vi "CalculateBPM.vi"(11 "Raw Beam Profile":dbl[][](array[numeric]) format="%0.2f") -> (3 "BPM":cluster{dbl[], "Beam Profile":dbl[]}[](array[cluster]))   [LabVIEW 2012]
uses:
  <vilib>/Analysis/_algsub.llb/Vector Norm Type.ctl
  <vilib>/Analysis/baseanly.llb/Normalize Vector.vi
  <vilib>/Analysis/baseanly.llb/Unit Vector (DBL).vi
  <vilib>/Analysis/NI_AALPro.lvlib
  <vilib>/Analysis/NI_AALBase.lvlib
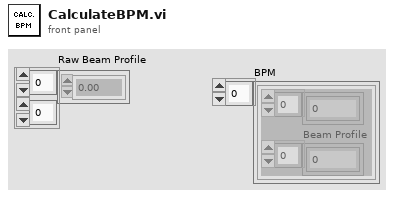
[diagram p1: front panel]
types:
  T1 = typedef "NI_AALPro.lvlib/Vector Norm Type.ctl" = u16
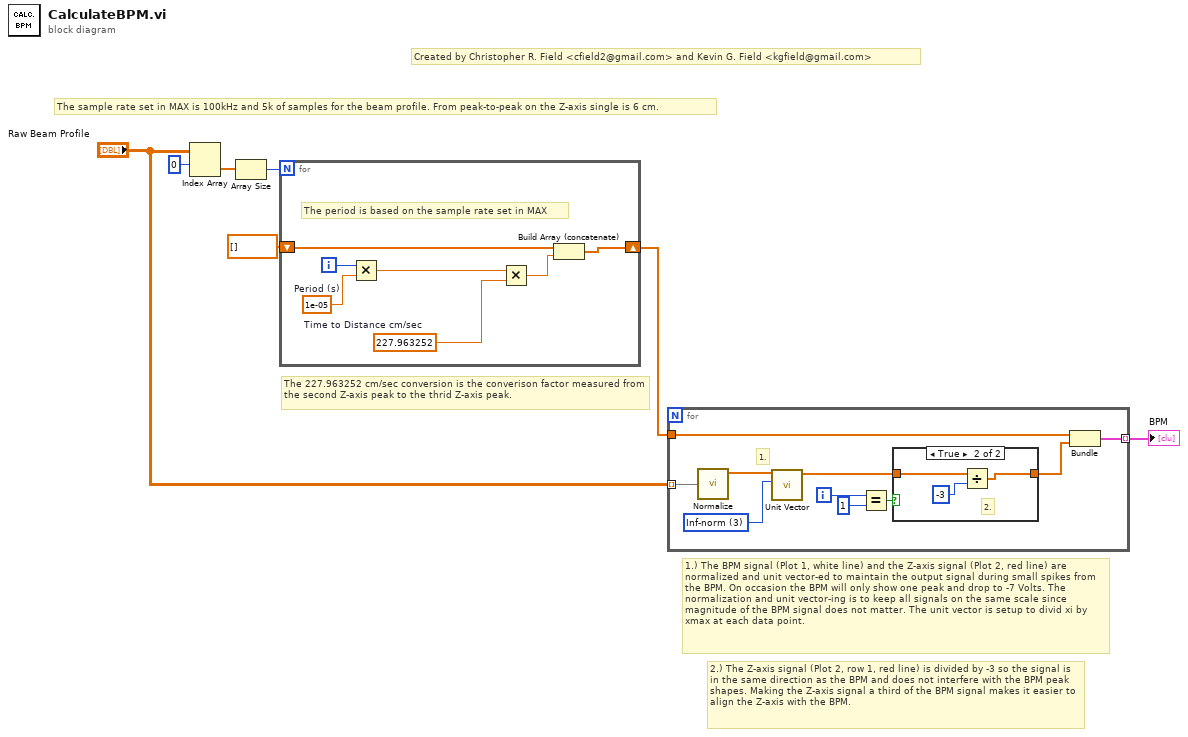
[diagram p0: block diagram]
diagram:
  # "Created by Christopher R. Field <cfield2@gmail.com> and Kevin G. Field <kgfield@gmail.com>"
  # "1.) The BPM signal (Plot 1, white line) and the Z-axis signal (Plot 2, red line) are normalized and unit vector-ed to maintain the output signal during small spikes from the BPM. On occasion the BPM will only show one peak and drop to -7 Volts. The normalization and unit vector-ing is to keep all signals on the same scale since magnitude of the BPM signal does not matter. The unit vector is setup to divid xi by xmax at each data point."
  # "2.) The Z-axis signal (Plot 2, row 1, red line) is divided by -3 so the signal is in the same direction as the BPM and does not interfere with the BPM peak shapes. Making the Z-axis signal a third of the BPM signal makes it easier to align the Z-axis with the BPM."
  # "The 227.963252 cm/sec conversion is the converison factor measured from the second Z-axis peak to the thrid Z-axis peak."
  # "The sample rate set in MAX is 100kHz and 5k of samples for the beam profile. From peak-to-peak on the Z-axis single is 6 cm."
  n1 = Index Array(array="Raw Beam Profile", index (row)=0) -> (element=w5:dbl[])  [unwired: 1 in]
  n2 = Array Size(array=w5) -> (size(s)=w4:i32)
  n3 = for {
    N: w4 -> [_]
    shift-right: [w14] -> w2
    shift-left: dbl[] [] -> [w11]
    i -> [w12]
    w8 = 227.963252  # Time to Distance cm/sec
    w13 = 1e-05  # Period (s)
    # "The period is based on the sample rate set in MAX"
    n4 = Multiply(x=w12, y=w13) -> (x*y=w10:dbl)
    n5 = Multiply(x=w10, y=w8) -> (x*y=w9:dbl)
    n6 = Build Array (concatenate)(w11, w9) -> (w14:dbl[])
  }
  n7 = for {
    tunnel: "Raw Beam Profile" -> [w19] mode=indexing
    tunnel: w2 -> [w24]
    tunnel: [w23] -> w1 mode=indexing
    i -> [w22]
    w17 = T1 3 items=["1-norm"=1, "2-norm"=2, "Inf-norm"=3, "-Inf-norm"=4, "User Defined"=5] ("norm type")
    # "1."
    n8 = call-poly <vilib>:"Normalize.vi"("Vector"=w19) -> ("Normalized Vector"=w18:dbl[])  [unwired: 1 in, 3 out]
    n9 = call-poly <vilib>:"Unit Vector.vi"("norm type"=w17, "Input Vector"=w18) -> ("Unit Vector"=w16:dbl[])  [unwired: 7 in, 2 out]
    n10 = Equal?(x=w22, y=1) -> (x = y?=w20:bool)
    n11 = case shown="True" w20 {
      tunnel: [w25 w26] -> w15
      tunnel: w16 -> [w25 w27]
      frame False {
      }
      frame True {
        # "2."
        n12 = Divide(x=w27, y=-3) -> (x/y=w26:dbl[])
      }
    }
    n13 = Bundle(w24, "Unit Vector"=w15) -> (w23:cluster{dbl[], "Unit Vector":dbl[]})  [unwired: 1 in]
  }
  "BPM" <- w1
